vi "Remember_RD_Folders.vi"(1 "Empty list":bool, 2 "Folders to Remember":path) -> (0 "List of Folders":path[](array[path]))   [LabVIEW 2010]
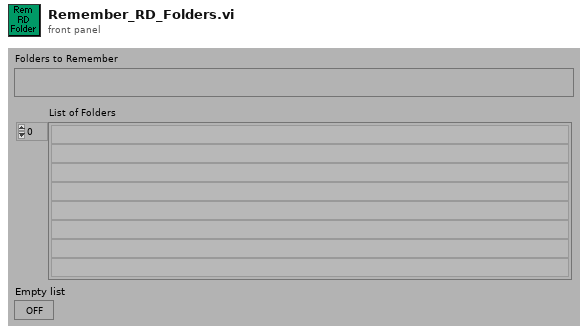
[diagram p1: front panel]
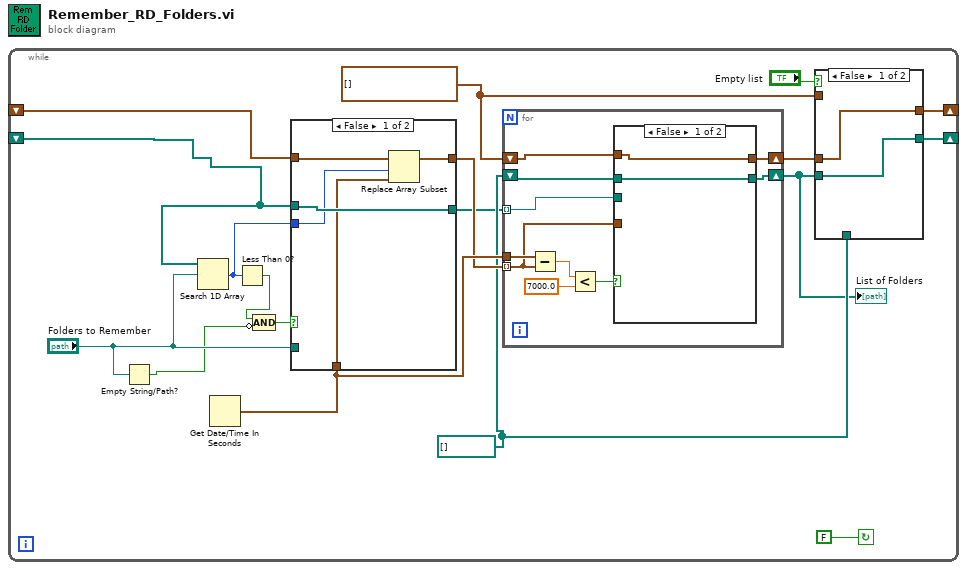
[diagram p0: block diagram]
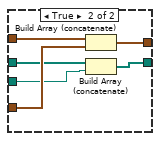
[diagram p2: hidden frame]
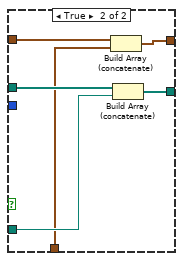
[diagram p4: hidden frame]
diagram:
  n1 = while {
    shift-left: _ -> [w17]
    shift-right: [w5] -> _
    shift-right: [w7] -> _
    shift-left: _ -> [w11]
    stop <- FALSE continue-if-true
    w8 = timestamp[] []
    w6 = path[] []
    n2 = Empty String/Path?(string/path="Folders to Remember") -> (empty?=w13:bool)
    n3 = Search 1D Array(1D array=w17, element="Folders to Remember") -> (index of element=w1:i32)  [unwired: 1 out]
    n4 = Get Date/Time In Seconds() -> (seconds since 1Jan1904=w10:timestamp)
    n5 = Less Than 0?(x=w1) -> (x < 0?=w14:bool)
    n6 = Compound Arithmetic op=AND(w14, invert w13) -> (w15:bool)
    n7 = case shown="False" w15 {
      tunnel: w17 -> [w45 w51]
      tunnel: "Folders to Remember" -> [_ w50]
      tunnel: [w45 w49] -> w2
      tunnel: w11 -> [w44 w48]
      tunnel: [w43 w47] -> w9
      tunnel: w10 -> [w41 w46]
      tunnel: w1 -> [w42 _]
      frame False {
        n8 = Replace Array Subset(array=w44, new element=w41, index=w42) -> (w43:timestamp[])
      }
      frame True {
        n9 = Build Array (concatenate)(w48, w46) -> (w47:timestamp[])
        n10 = Build Array (concatenate)(w51, w50) -> (w49:path[])
      }
    }
    n11 = for {
      shift-right: [w22] -> w4
      shift-left: w8 -> [w23]
      shift-right: [w20] -> w3
      shift-left: w6 -> [w21]
      tunnel: w10 -> [w26]
      tunnel: w9 -> [w24] mode=indexing
      tunnel: w2 -> [w19] mode=indexing
      n12 = Subtract(x=w26, y=w24) -> (x-y=w28:dbl)
      n13 = Less?(x=w28, y=7000.0) -> (x < y?=w25:bool)
      n14 = case shown="False" w25 {
        tunnel: w24 -> [_ w36]
        tunnel: w23 -> [w30 w35]
        tunnel: [w30 w34] -> w22
        tunnel: w21 -> [w29 w33]
        tunnel: [w29 w32] -> w20
        tunnel: w19 -> [_ w31]
        frame False {
        }
        frame True {
          n15 = Build Array (concatenate)(w35, w36) -> (w34:timestamp[])
          n16 = Build Array (concatenate)(w33, w31) -> (w32:path[])
        }
      }
    }
    "List of Folders" <- w3
    n17 = case shown="False" "Empty list" {
      tunnel: w8 -> [_ w40]
      tunnel: [w37 w40] -> w7
      tunnel: w6 -> [_ w39]
      tunnel: [w38 w39] -> w5
      tunnel: w3 -> [w38 _]
      tunnel: w4 -> [w37 _]
      frame False {
      }
      frame True {
      }
    }
  }
